vi "Verify.vi"(8 "error in (no error)":errorcluster, 10 "Mock.lvclass":refnum<class "Mock.lvclass">, 11 "LUnit Test Case In":refnum<class "Test Case.lvclass">) -> (0 "error out":errorcluster, 3 "LUnit Test Case Out":refnum<class "Test Case.lvclass">)   [LabVIEW 2020, in "Verifier.lvclass"]
uses:
  Validator/Verifier.lvclass
  <vilib>/Astemes/LUnit/Test Case.lvclass
  Mock/Mock.lvclass
  <vilib>/Astemes/LUnit/Test Case.lvclass/Test Case.ctl
  <vilib>/Astemes/LUnit/Append Fail Result.vi
  <vilib>/Astemes/LUnit/Append Pass Result.vi
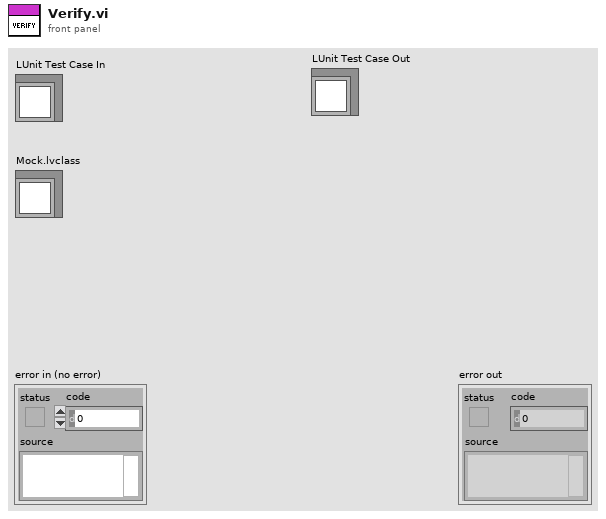
[diagram p1: front panel]
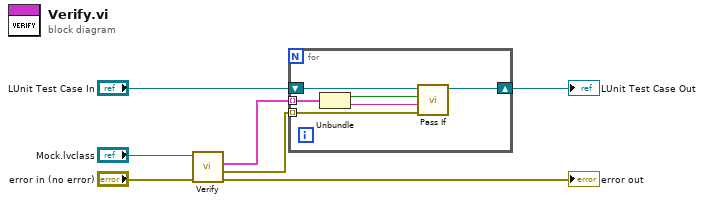
[diagram p0: block diagram]
diagram:
  n1 = call "Verify.vi"("error in (no error)"="error in (no error)", "Mock in"="Mock.lvclass") -> ("error out"=→"error out":errorcluster, "Errors"=w2:errorcluster[], "Results"=w3:cluster{"Passed?":bool, "Message":string}[])  [unwired: 7 in]
  n2 = for {
    shift-right: [w12] -> w6
    shift-left: "LUnit Test Case In" -> [w13]
    tunnel: w3 -> [w10] mode=indexing
    tunnel: w2 -> [w11] mode=indexing
    n3 = Unbundle(w10) -> ("Passed?"=w9:bool, "Message"=w8:string)
    n4 = call <vilib>:"Pass If.vi"("error in (no error)"=w11, "Message"=w8, "Pass?"=w9, "LUnit Test Case In"=w13) -> ("LUnit Test Case Out"=w12:refnum<class "Test Case.lvclass">)  [unwired: 6 in, 1 out]
  }
  "LUnit Test Case Out" <- w6
